vi "Simple Document Creation Example.vi"() -> ()   [LabVIEW 2017]
uses:
  <vilib>/printing/ReportDocExtensions.llb/File_types_for_reports.ctl
  <vilib>/BenjaminR/LabVIEW NPOI/LabVIEW NPOI/Document/Append Table (double).vi
  <vilib>/BenjaminR/LabVIEW NPOI/LabVIEW NPOI/Document/Document.lvclass
  <vilib>/Utility/NIReport.llb/NI_ReportGenerationCore.lvlib
panel:
  in  "Relative Humidity":dbl[][](array[numeric])=[[0.54, 0.65, 0.56, 0.5, 0.45]]
  in  "Month":string[](array[string])=["Jan", "Feb", "Mar", "Apr", "May"]
  in  "File Path":path
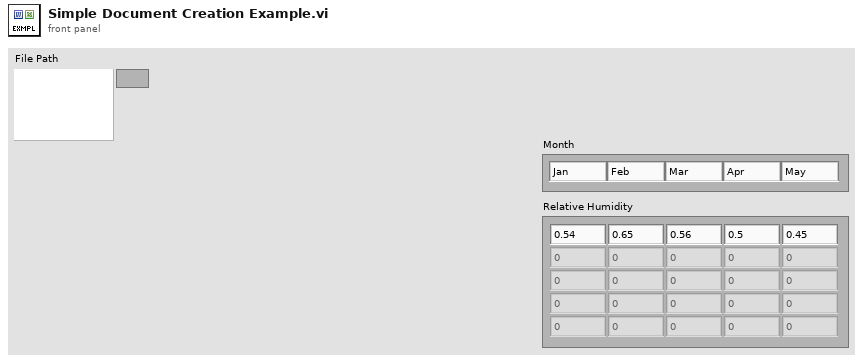
[diagram p1: front panel]
types:
  T1 = typedef "NI_ReportGenerationCore.lvlib/File_types_for_reports.ctl" = enum16{".jpg", ".png", ".html", ".gif"}
  T2 = typedef "imagedata.ctl" = cluster{"image type":i32, "image depth":i32, "image":u8[], "mask":u8[], "colors":u32[], "Rectangle":cluster{"left":i16, "top":i16, "right":i16, "bottom":i16}}
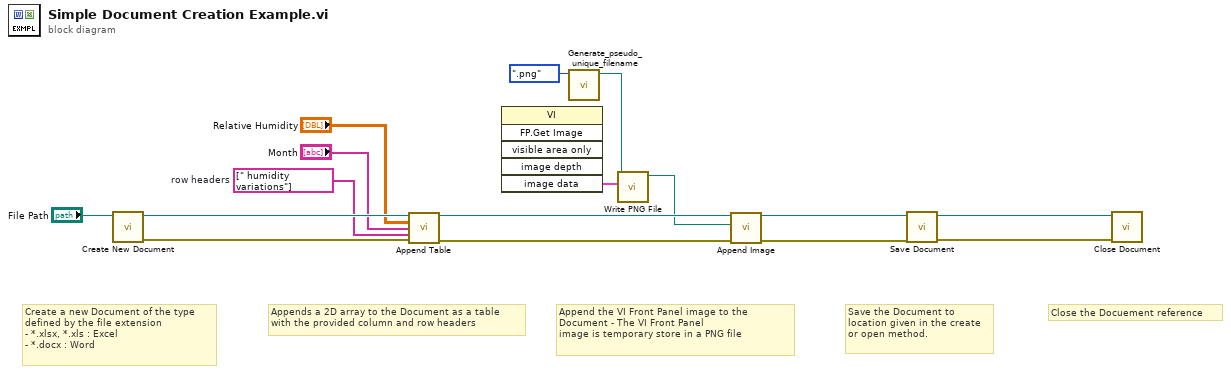
[diagram p0: block diagram]
diagram:
  w11 = string[] [" humidity variations"]  # row headers
  # "Close the Docuement reference"
  # "Save the Document to location given in the create or open method."
  # "Append the VI Front Panel image to the Document - The VI Front Panel\nimage is temporary store in a PNG file"
  # "Appends a 2D array to the Document as a table \nwith the provided column and row headers"
  # "Create a new Document of the type\ndefined by the file extension\n- *.xlsx, *.xls : Excel\n- *.docx : Word"
  n1 = call <vilib>:"Create New Document.vi"("File Path"="File Path") -> ("error out"=w14:errorcluster, "Document out"=w15:refnum<class "Document.lvclass">)  [unwired: 9 in]
  n2 = call-poly <vilib>:"Append Table.vi"("Document in"=w15, "Table"="Relative Humidity", "Column Headers"="Month", "Row Headers"=w11, "error in (no error)"=w14) -> ("Document out"=w10:refnum<class "Document.lvclass">, "error out"=w9:errorcluster)  [unwired: 9 in]
  n3 = invoke class="VI" method="FP.Get Image"() -> ("image data"=w8:T2)  [unwired: 6 in, 5 out]
  n4 = call <vilib>:"Generate_pseudo_unique_filename.vi"("file type(.jpg)"=File_types_for_reports.".png") -> ("generated path"=w6:path)  [unwired: 8 in, 2 out]
  n5 = call <vilib>:"Write PNG File.vi"("image data"=w8, "path to PNG file"=w6) -> ("path"=w5:path)  [unwired: 8 in, 1 out]
  n6 = call <vilib>:"Append Image.vi"("error in (no error)"=w9, "Image File Path"=w5, "Document in"=w10) -> ("error out"=w3:errorcluster, "Document out"=w4:refnum<class "Document.lvclass">)  [unwired: 7 in]
  n7 = call <vilib>:"Save Document.vi"("error in (no error)"=w3, "Document in"=w4) -> ("error out"=w2:errorcluster, "Document out"=w1:refnum<class "Document.lvclass">)  [unwired: 8 in]
  n8 = call <vilib>:"Close Document.vi"("error in (no error)"=w2, "Document in"=w1) -> ()  [unwired: 9 in, 1 out]
